vi "Temperature_FGV.vi"(7 "Command":enum16{"SET", "GET"}(ring), 8 "error in (no error)":errorcluster, 11 "Temperature_IN":dbl) -> (0 "error out":errorcluster, 3 "Temperature_OUT":dbl)   [LabVIEW 2017]
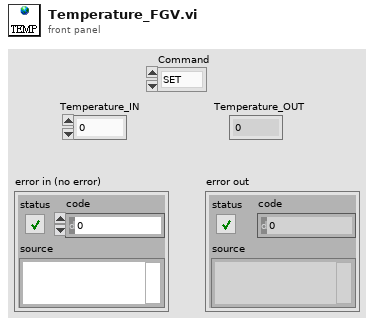
[diagram p1: front panel]
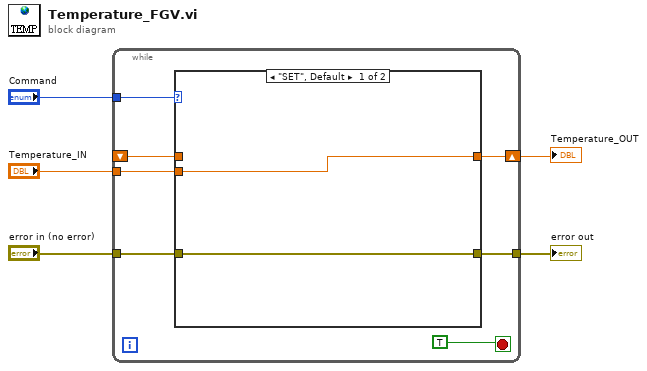
[diagram p0: block diagram]
diagram:
  n1 = while {
    tunnel: "Command" -> [w12]
    shift-right: [w11] -> w4
    shift-left: _ -> [w9]
    tunnel: "Temperature_IN" -> [w10]
    tunnel: [w7] -> w2
    tunnel: "error in (no error)" -> [w6]
    stop <- TRUE stop-if-true
    n2 = case shown="\"SET\", Default" w12 {
      tunnel: [w14 w16] -> w11
      tunnel: w10 -> [w14 _]
      tunnel: w9 -> [_ w16]
      tunnel: [w13 w15] -> w7
      tunnel: w6 -> [w13 w15]
      frame "SET", Default {
      }
      frame "GET" {
      }
    }
  }
  "Temperature_OUT" <- w4
  "error out" <- w2
